vi "Write Conveyor.vi"(8 "error in (no error)":errorcluster, 10 "Conveyor":refnum<k20>, 11 "ODESimulator_Base_Conveyor in":refnum<class "ODESimulator_Base_Conveyor.lvclass">) -> (0 "error out":errorcluster, 3 "ODESimulator_Base_Conveyor out":refnum<class "ODESimulator_Base_Conveyor.lvclass">)   [LabVIEW 2017, in "NI_Robotics_Simulator.lvlib" / "ODESimulator_Base_Conveyor.lvclass"]
uses:
  <vilib>/robotics/Simulator/Robot Factory/Conveyor/Base/ODESimulator_Base_Conveyor.lvclass
  <vilib>/robotics/Simulator/Robot Factory/Conveyor/Base/ODESimulator_Base_Conveyor.lvclass/ODESimulator_Base_Conveyor.ctl
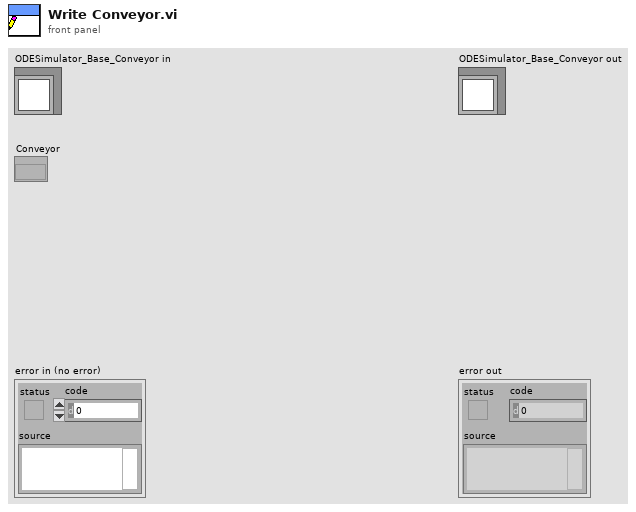
[diagram p1: front panel]
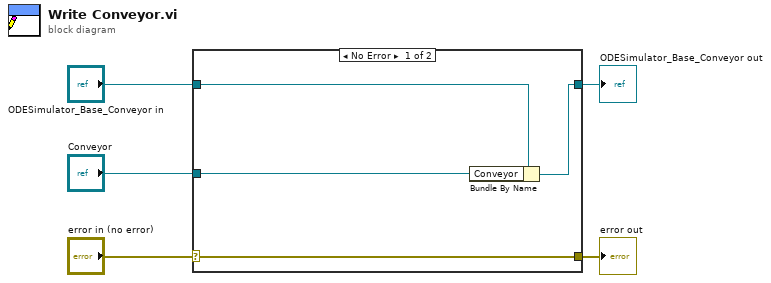
[diagram p0: block diagram]
diagram:
  n1 = case shown="No Error" "error in (no error)" {
    selector: "error in (no error)" -> [w9 w10]
    tunnel: [w9 w10] -> w4
    tunnel: [w7 w11] -> w2
    tunnel: "ODESimulator_Base_Conveyor in" -> [w8 w11]
    tunnel: "Conveyor" -> [w6 _]
    frame No Error {
      n2 = Bundle By Name(cluster=w8, "Conveyor"=w6) -> (w7:refnum<class "ODESimulator_Base_Conveyor.lvclass">)
    }
    frame Error {
    }
  }
  "error out" <- w4
  "ODESimulator_Base_Conveyor out" <- w2
